vi "ORS_DrawFlattenedPixmap8.vi"(6 "colormap data string":string, 7 "height":i16, 8 "width":i16, 9 "image data":u8[](array[numeric])) -> (3 "new picture":picture)   [LabVIEW 2024]
doc: "Draws a 1-, 4-, or 8-bit pixmap or a 24-bit RGB pixmap into a picture."
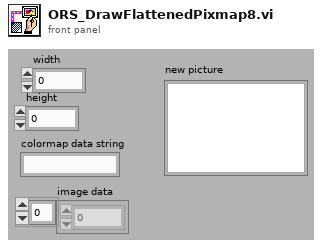
[diagram p1: front panel]
types:
  T1 = cluster{"left":i16, "left":i16, "height":i16, "width":i16}
  T2 = cluster{"default foreground":u32, "default background":u32}
  T3 = cluster{"opcode-Copy Pixmap":i16, i32, i32, cluster{"left":i16, "left":i16, "height":i16, "width":i16}, i16, cluster{"default foreground":u32, "default background":u32}}
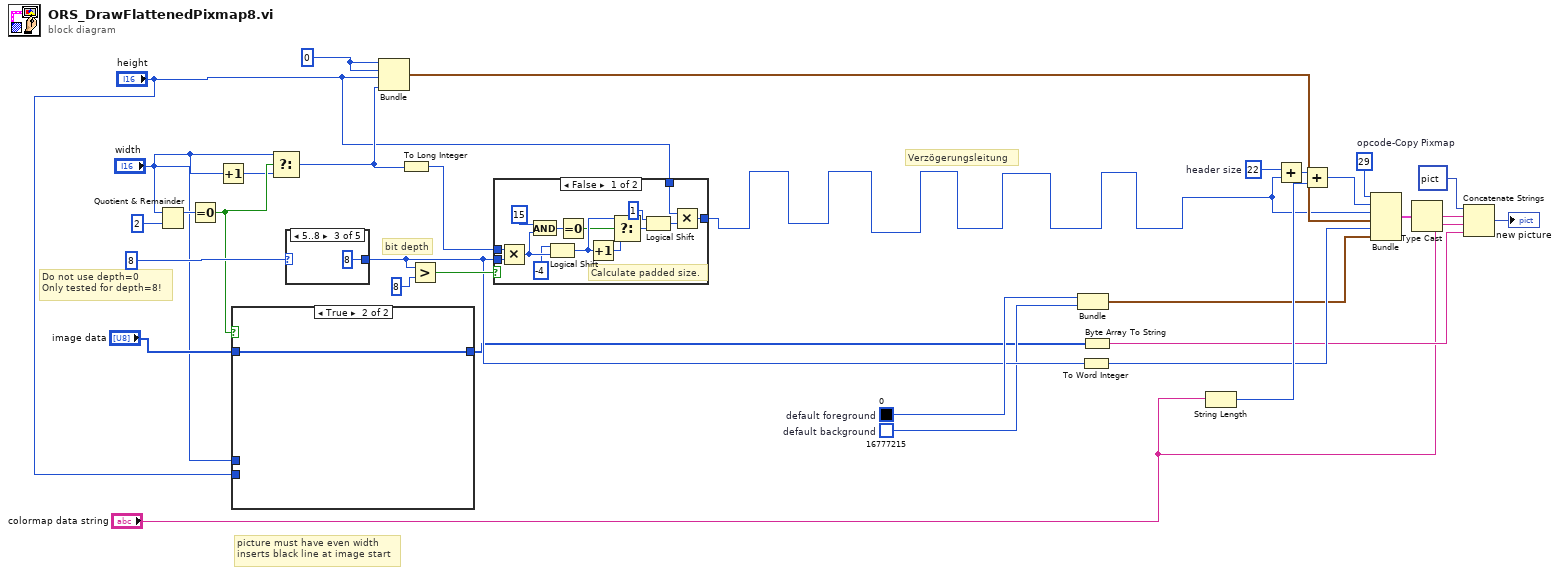
[diagram p0: block diagram]
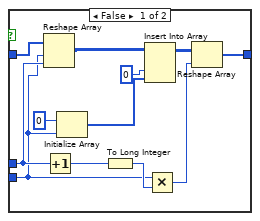
[diagram p2: hidden frame]
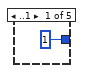
[diagram p3: hidden frame]
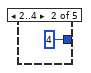
[diagram p4: hidden frame]
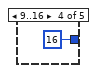
[diagram p5: hidden frame]
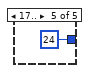
[diagram p6: hidden frame]
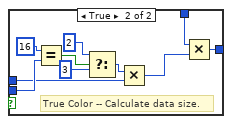
[diagram p7: hidden frame]
diagram:
  w11 = i16 0 ("left")
  w24 = u32 16777215  # default background
  w26 = u32 0  # default foreground
  w16 = i16 22  # header size
  w14 = i16 29  # opcode-Copy Pixmap
  # "picture must have even width\ninserts black line at image start"
  # "Verzögerungsleitung"
  # "Do not use depth=0\nOnly tested for depth=8!"
  # "bit depth"
  n1 = Quotient & Remainder(x="width", y=2) -> (x-y*floor(x/y)=w8:i32)  [unwired: 1 out]
  n2 = Equal To 0?(x=w8) -> (x = 0?=w6:bool)
  n3 = Increment(x="width") -> (x+1=w5:i16)
  n4 = case shown="True" w6 {
    tunnel: "image data" -> [w44 w45]
    tunnel: [w42 w45] -> w3
    tunnel: "height" -> [w33 _]
    tunnel: "width" -> [w34 _]
    frame False {
      n5 = Reshape Array(w44, w33, w34) -> (w35:u8[][])
      n6 = Increment(x=w34) -> (x+1=w40:i16)
      n7 = Initialize Array(u8 0 ("left"), w33) -> (w38:u8[])
      n8 = To Long Integer(number=w40) -> (32bit integer=w39:i32)
      n9 = Insert Into Array(array=w35, index (col)=0 ("disabled index (col)"), new element=w38) -> (w36:u8[][])  [unwired: 1 in]
      n10 = Multiply(x=w33, y=w39) -> (x*y=w41:i32)
      n11 = Reshape Array(w36, w41) -> (w42:u8[])
    }
    frame True {
    }
  }
  n12 = Select(t="width", s=w6, f=w5) -> (s? t:f=w4:i16)
  n13 = case shown="5..8" 8 ("image depth") {
    tunnel: [1 4 8 16 24] -> w25
    frame ..1 {
    }
    frame 2..4 {
    }
    frame 5..8 {
    }
    frame 9..16 {
    }
    frame 17.. {
    }
  }
  n14 = Bundle("left"=w11, "left"=w11, "height"="height", "width"=w4) -> (w21:T1)  [unwired: 1 in]
  n15 = To Long Integer(number=w4) -> (32bit integer=w20:i32)
  n16 = Greater?(x=w25, y=u8 8) -> (0:w27:bool)
  n17 = case shown="False" w27 {
    tunnel: [w64 w74] -> w10
    tunnel: "height" -> [w60 w73]
    tunnel: w25 -> [w52 w71]
    tunnel: w20 -> [w51 w69]
    frame False {
      # "Calculate padded size."
      n18 = Multiply(x=w51, y=w52) -> (x*y=w54:i32)
      n19 = And(x=15, y=w54) -> (x .and. y?=w56:i32)
      n20 = Logical Shift(y=-4, x=w54) -> (x << y=w58:i32)
      n21 = Equal To 0?(x=w56) -> (x = 0?=w57:bool)
      n22 = Increment(x=w58) -> (x+1=w59:i32)
      n23 = Select(t=w58, s=w57, f=w59) -> (s? t:f=w62:i32)
      n24 = Logical Shift(y=1, x=w62) -> (x << y=w63:i32)
      n25 = Multiply(x=w60, y=w63) -> (x*y=w64:i32)
    }
    frame True {
      # "True Color -- Calculate data size."
      n26 = Equal?(x=16, y=w71) -> (x = y?=w68:bool)
      n27 = Select(t=2, s=w68, f=3) -> (s? t:f=w65:i32)
      n28 = Multiply(x=w65, y=w69) -> (x*y=w72:i32)
      n29 = Multiply(x=w73, y=w72) -> (x*y=w74:i32)
    }
  }
  n30 = Bundle("default foreground"=w26, "default background"=w24) -> (w29:T2)  [unwired: 1 in]
  n31 = To Word Integer(number=w25) -> (16bit integer=w31:i16)
  n32 = Byte Array To String(unsigned byte array=w3) -> (string=w30:string)
  n33 = String Length(string="colormap data string") -> (length=w32:i32)
  n34 = Add(x=w16, y=w10) -> (x+y=w17:i32)
  n35 = Add(x=w17, y=w32) -> (x+y=w18:i32)
  n36 = Bundle "Bundle"("opcode-Copy Pixmap"=w14, w18, w10, w21, w31, w29) -> (w15:T3)  [unwired: 1 in]
  n37 = Type Cast(x=w15) -> (*(type *) &x=w19:string)  [unwired: 1 in]
  n38 = Concatenate Strings(picture data[5B] ("picture"), w19, "colormap data string", w30) -> (→"new picture":picture)
